vi "ConvertDesiredRefreshRatio.vi"(1 "Desired Refresh Ratio":dbl) -> (0 "Required Number of Pump Iterations":dbl)   [LabVIEW 2016]
uses:
  CurrentSwitchValues_GlobalVariable.vi
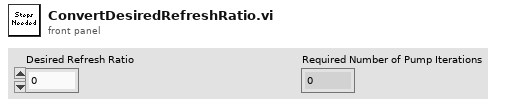
[diagram p1: front panel]
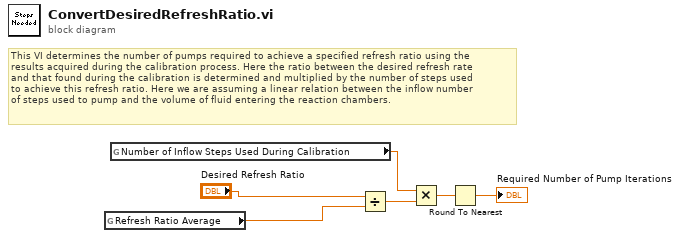
[diagram p0: block diagram]
diagram:
  # "This VI determines the number of pumps required to achieve a specified refresh ratio using the \nresults acquired during the calibration process. Here the ratio between the desired refresh rate \nand that found during the calibration is determined and multiplied by the number of steps used\nto achieve this refresh ratio. Here we are assuming a linear relation between the inflow number \nof steps used to pump and the volume of fluid entering the reaction chambers."
  n1 = global read "CurrentSwitchValues_GlobalVariable.vi" "Refresh Ratio Average"() -> (w1:dbl)
  n2 = global read "CurrentSwitchValues_GlobalVariable.vi" "Number of Inflow Steps Used During Calibration"() -> (w2:dbl)
  n3 = Divide(x="Desired Refresh Ratio", y=w1) -> (x/y=w5:dbl)
  n4 = Multiply(x=w2, y=w5) -> (x*y=w4:dbl)
  n5 = Round To Nearest(number=w4) -> (nearest integer value=→"Required Number of Pump Iterations":dbl)
